vi "websocket test.vi"() -> ()   [LabVIEW 2019]
uses:
  <vilib>/MediaMongrels Ltd/WebSockets/WebSockets/WebSocket/WebSocket.lvclass/WebSocket.ctl
  <vilib>/MediaMongrels Ltd/WebSockets/WebSockets/WebSocket Server/WebSocket Server.lvclass/WebSocket Server.ctl
  <vilib>/MediaMongrels Ltd/WebSockets/WebSockets/WebSocket/Read Return Headers.vi
  <vilib>/MediaMongrels Ltd/WebSockets/WebSockets/WebSocket Server/Read Request URI.vi
  <vilib>/MediaMongrels Ltd/WebSockets/WebSockets/WebSocket Server/WebSocket Server.lvclass
  C:/Program Files (x86)/National Instruments/LabVIEW 2019/vi.lib/MediaMongrels Ltd/WebSockets/WebSockets/WebSocket/WebSocket.lvclass
  <vilib>/MediaMongrels Ltd/WebSockets/Sockets/VISA TCP Listener/VISA TCP Listener.lvclass
  <vilib>/ptbypt/NI_PtbyPt.lvlib
panel:
  in  "Send":bool
  in  "Data":string
  out "Received Data":string
  out "HTTP Headers":variant
  out "Request URI":string
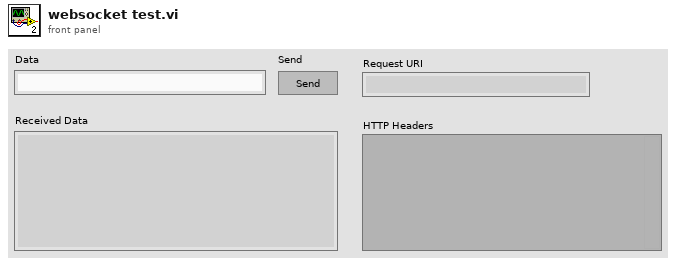
[diagram p1: front panel]
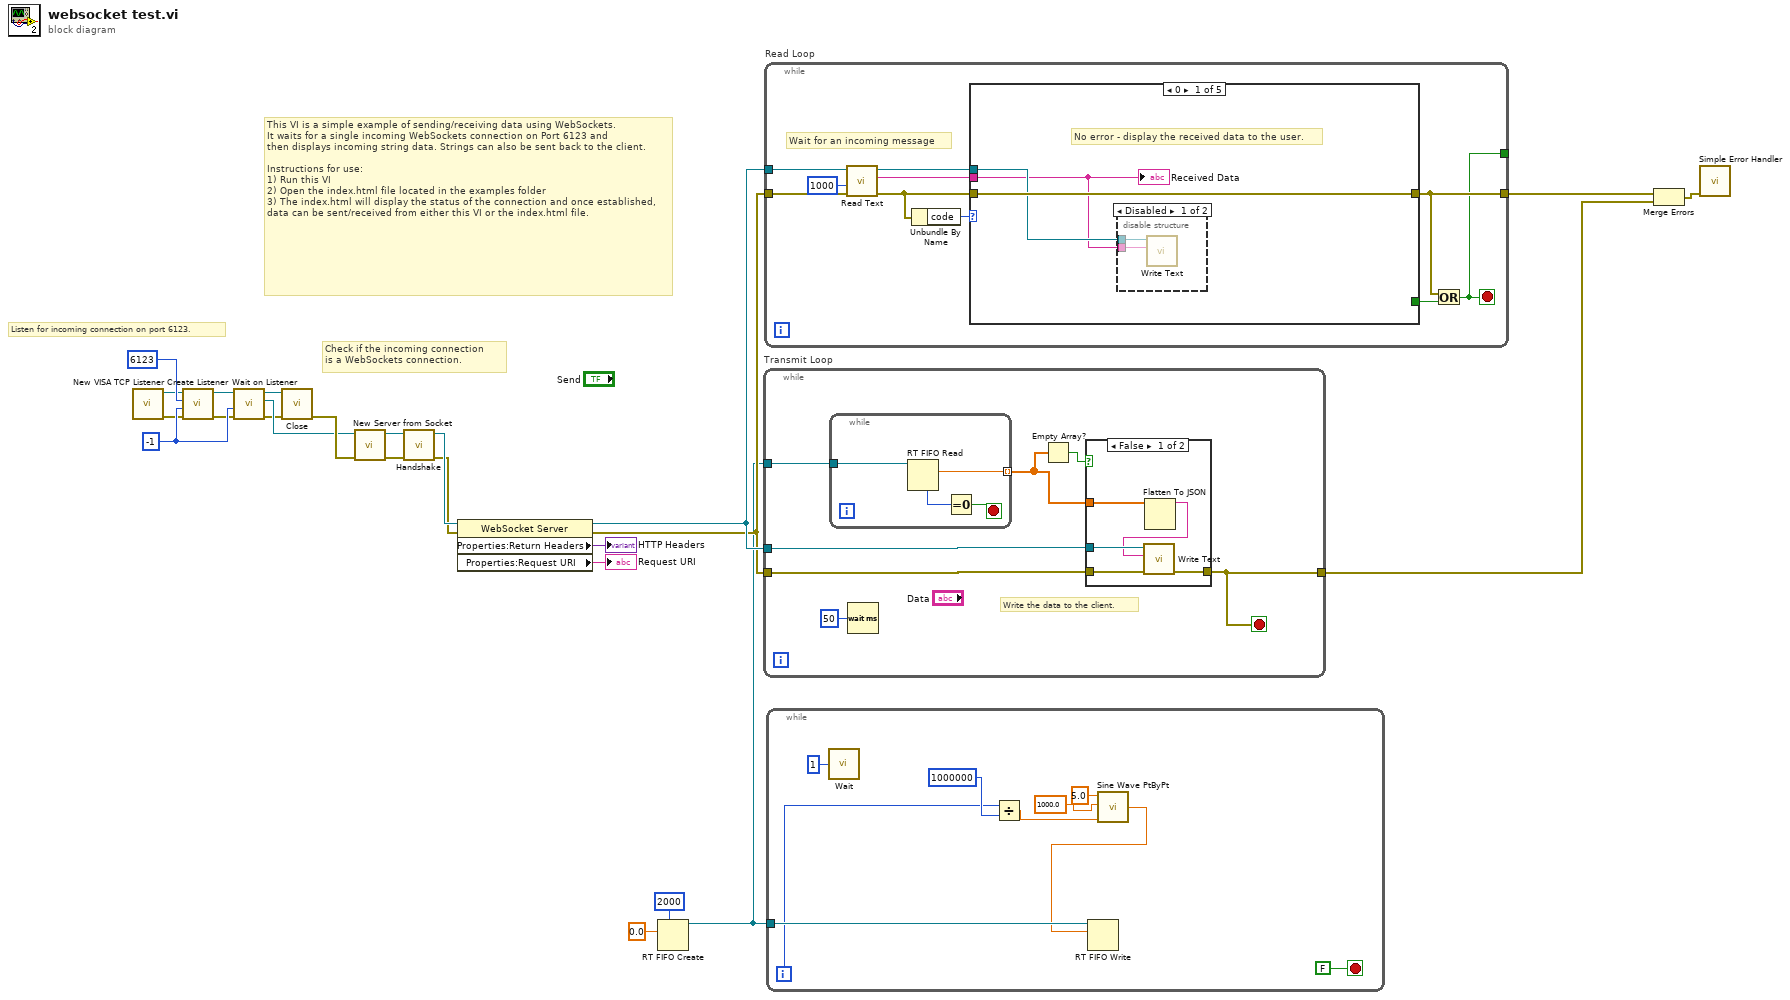
[diagram p0: block diagram]
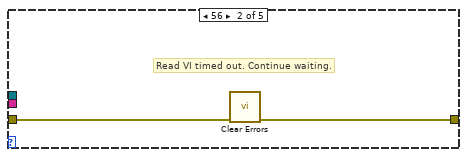
[diagram p3: hidden frame]
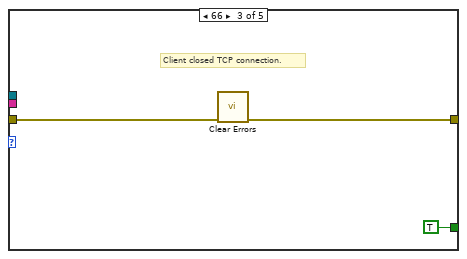
[diagram p4: hidden frame]
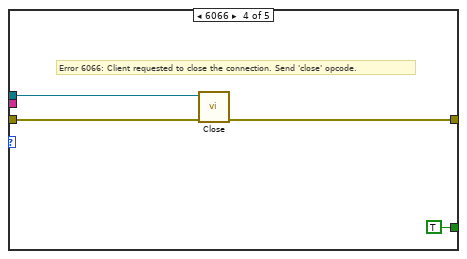
[diagram p5: hidden frame]
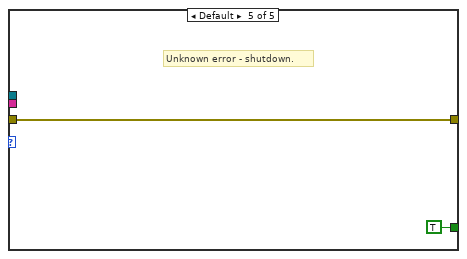
[diagram p6: hidden frame]
diagram:
  w22 = -1 ("timeout ms (25000)")
  # "This VI is a simple example of sending/receiving data using WebSockets.\nIt waits for a single incoming WebSockets connection on Port 6123 and\nthen displays incoming string data. Strings can also be sent back to the client.\n\nInstructions for use:\n1) Run this VI\n2) Open the index.html file located in the examples folder\n3) The index.html will display the status of the connection and once established, data can be sent/received from either this VI or the index.html file."
  # "Check if the incoming connection\nis a WebSockets connection."
  # "Listen for incoming connection on port 6123."
  n1 = call <vilib>:"New VISA TCP Listener.vi"() -> ("error out"=w16:errorcluster, "VISA TCP Listener out"=w15:refnum<class "VISA TCP Listener.lvclass">)  [unwired: 10 in]
  n2 = call-dynamic "Create Listener.vi"("error in (no error)"=w16, "timeout ms (5000)"=w22, "Port"=u16 6123 ("port"), "VISA TCP Listener in"=w15) -> ("error out"=w18:errorcluster, "VISA TCP Listener out"=w20:refnum<class "VISA TCP Listener.lvclass">)  [unwired: 6 in]
  n3 = call-dynamic "Wait on Listener.vi"("error in (no error)"=w18, "timeout ms (5000)"=w22, "VISA TCP Listener in"=w20) -> ("error out"=w17:errorcluster, "Socket out"=w23:refnum<class "Socket.lvclass">, "VISA TCP Listener out"=w19:refnum<class "VISA TCP Listener.lvclass">)  [unwired: 6 in]
  n4 = call-dynamic "Close.vi"("error in (no error)"=w17, "VISA TCP Listener in"=w19) -> ("error out"=w24:errorcluster)  [unwired: 9 in]
  n5 = call <vilib>:"New Server from Socket.vi"("error in (no error)"=w24, "Socket"=w23) -> ("error out"=w9:errorcluster, "WebSocket Server out"=w8:refnum<class "WebSocket Server.lvclass">)  [unwired: 8 in]
  n6 = call-dynamic "Handshake.vi"("error in (no error)"=w9, "WebSocket Connection in"=w8) -> ("error out"=w7:errorcluster, "WebSocket Connection out"=w11:refnum<class "WebSocket Server.lvclass">)  [unwired: 8 in]
  n7 = property class="WebSocket Server"(reference=w11, error in=w7) -> (reference out=w12:refnum<class "WebSocket Server.lvclass">, error out=w10:errorcluster, "Properties:Return Headers"=→"HTTP Headers":variant, "Properties:Request URI"=→"Request URI":string)
  n8 = RT FIFO Create(1:0.0, 4:u32 2000 ("size (10)")) -> (8:w3:refnum<k33>)  [unwired: 6 in, 2 out]
  n9 = while "Transmit Loop" {
    tunnel: w12 -> [w31]
    tunnel: [w30] -> w4
    tunnel: w10 -> [w29]
    tunnel: w3 -> [w28]
    stop <- w30 stop-if-true
    # "Write the data to the client."
    n10 = while {
      tunnel: w28 -> [w41]
      tunnel: [w40] -> w26 mode=indexing
      stop <- w38 stop-if-true
      n11 = RT FIFO Read(0:w41) -> (7:w39:u32, 9:w40:dbl)  [unwired: 3 in, 3 out]
      n12 = Equal To 0?(x=w39) -> (x = 0?=w38:bool)
    }
    n13 = Wait (ms)(milliseconds to wait=u32 50) -> ()  [unwired: 1 out]
    n14 = Empty Array?(array=w26) -> (empty?=w25:bool)
    n15 = case shown="False" w25 {
      tunnel: w31 -> [w36 _]
      tunnel: [w35 w37] -> w30
      tunnel: w29 -> [w34 w37]
      tunnel: w26 -> [w32 _]
      frame False {
        n16 = Flatten To JSON(anything=w32) -> (JSON string=w33:string)  [unwired: 2 in, 1 out]
        n17 = call-dynamic "Write Text.vi"("error in (no error)"=w34, "String Data"=w33, "WebSocket in"=w36) -> ("error out"=w35:errorcluster)  [unwired: 7 in, 1 out]
      }
      frame True {
      }
    }
  }
  n18 = while "Read Loop" {
    tunnel: w12 -> [w51]
    tunnel: [w42] -> _
    tunnel: [w44] -> w6
    tunnel: w10 -> [w45]
    stop <- w42 stop-if-true
    # "Wait for an incoming message"
    n19 = call-dynamic "Read Text.vi"("error in (no error)"=w45, "timeout ms (5000)"=1000 ("timeout ms (25000)"), "WebSocket in"=w51) -> ("error out"=w46:errorcluster, "Data"=w48:string, "WebSocket out"=w47:refnum<class "WebSocket Server.lvclass">)  [unwired: 6 in]
    n20 = Unbundle By Name(w46) -> ("code"=w49:i32)
    n21 = case shown="0" w49 {
      tunnel: w48 -> [w52 _ _ _ _]
      tunnel: [_ _ TRUE TRUE TRUE] -> w43
      tunnel: w47 -> [w53 _ _ w65 _]
      tunnel: w46 -> [w54 w58 w60 w63 w66]
      tunnel: [w54 w57 w59 w62 w66] -> w44
      frame 0 {
        # "No error - display the received data to the user."
        n22 = disable-structure shown="Disabled" {
          disable-tunnel: w53 -> [w56 _]
          disable-tunnel: w52 -> [w55 _]
          frame Disabled {
            n23 = call-dynamic "Write Text.vi"("String Data"=w55, "WebSocket in"=w56) -> ()  [unwired: 8 in, 2 out]
          }
          frame Enabled {
          }
        }
        "Received Data" <- w52
      }
      frame 56 {
        # "Read VI timed out. Continue waiting."
        n24 = call <vilib>:"Clear Errors.vi"("error in (no error)"=w58) -> ("error out"=w57:errorcluster)  [unwired: 5 in, 1 out]
      }
      frame 66 {
        # "Client closed TCP connection."
        n25 = call <vilib>:"Clear Errors.vi"("error in (no error)"=w60) -> ("error out"=w59:errorcluster)  [unwired: 5 in, 1 out]
      }
      frame 6066 {
        # "Error 6066: Client requested to close the connection. Send 'close' opcode."
        n26 = call-dynamic "Close.vi"("error in (no error)"=w63, "WebSocket in"=w65) -> ("error out"=w62:errorcluster)  [unwired: 9 in]
      }
      frame Default {
        # "Unknown error - shutdown."
      }
    }
    n27 = Or(x=w44, y=w43) -> (x .or. y?=w42:bool)
  }
  n28 = while {
    tunnel: w3 -> [w75]
    i -> [w68]
    stop <- FALSE stop-if-true
    n29 = call "Wait"("Count(mSec)"=u32 1 ("milliseconds to wait")) -> ()  [unwired: 1 out]
    n30 = Divide(x=w68, y=u32 1000000) -> (x/y=w70:dbl)
    n31 = call <vilib>:"Sine Wave PtByPt.vi"("time"=w70, "frequency"=1000.0, "amplitude"=5.0) -> ("sine wave"=w71:dbl)  [unwired: 1 in]
    n32 = RT FIFO Write(0:w75, 1:w71) -> ()  [unwired: 3 in, 4 out]
  }
  n33 = Merge Errors(w6, w4) -> (w5:errorcluster)
  n34 = call <vilib>:"Simple Error Handler.vi"("error in (no error)"=w5) -> ()  [unwired: 4 in, 5 out]
